vi "Calculate Optimiser Target Function.vi"(8 "error in (no error)":errorcluster, 10 "Observables":T1[](array[typedef]) {"Weight" min=0.0 max=1.0}, 11 "Analysis Framework":refnum<class "Analysis Framework.lvclass">) -> (0 "error out (no error)":errorcluster, 1 "Target":string, 2 "standard error":string, 3 "standard output":string, 4 "Error":bool, 5 "NaN":bool)   [LabVIEW 2020, in "Analysis Framework.lvclass"]
uses:
  Analysis Framework.lvclass
  Run Utilities/Optimiser Cell/Optimisation observable.ctl
  Run Utilities/Optimiser Cell/Optimiser Cell.lvclass
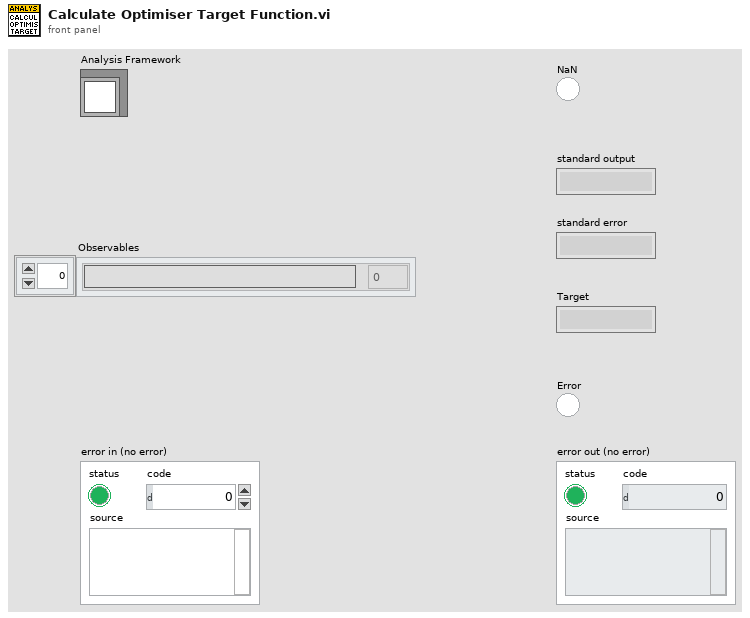
[diagram p1: front panel]
types:
  T1 = typedef "Run Utilities.lvlib/Optimiser Cell.lvclass/Optimisation observable.ctl" = cluster{"Name":string, "Weight":dbl}
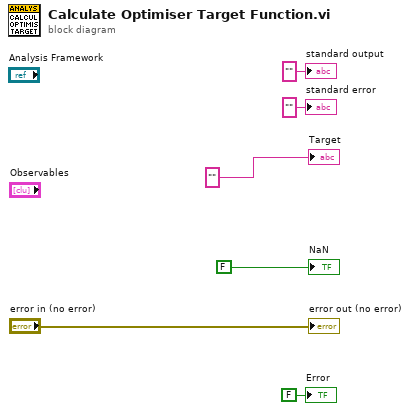
[diagram p0: block diagram]
diagram:
  "error out (no error)" <- "error in (no error)"
  "NaN" <- FALSE ("NaN")
  "Target" <- ""
  "standard output" <- "" ("standard output")
  "standard error" <- "" ("standard error")
  "Error" <- FALSE ("Error")
